vi "Main FPGA 5-axis with 1AxisLimit.vi"() -> ()   [LabVIEW 2013]
uses:
  <vilib>/Motion/MotorControl/_s/nism.interpretControlRegister.stateTransition.ctl
  <vilib>/Platform/TimedLoop/XDataNode/timing_clust.ctl
  <vilib>/Platform/TimedLoop/XDataNode/nitl_modes.ctl
  <vilib>/Platform/TimedLoop/XDataNode/wakeup.ctl
  <vilib>/Motion/MotorControl/_s/nism.digitalInputs.portA.ctl
  <vilib>/rvi/Emulation/niFpgaSctlEmulationGetInTimedLoop.vi
  <vilib>/rvi/Emulation/niFpgaEmulationReportErrorSimple.vi
  <vilib>/rvi/Emulation/niFpgaGetClockAttributes.vi
  <vilib>/rvi/Emulation/niFpgaCriticalErrorInLSC.vi
  Global FPGA.vi
  <vilib>/rvi/eio/common/nirviEmuTemplateMethod_errors.vi
  <vilib>/Motion/SoftMotion/Synchronization/nism.rioScan.generateSyncScan.vi
  <vilib>/rvi/Emulation/niFpgaProcessEmulError.vi
  <vilib>/Motion/MotorControl/_s/nism.interpretControlRegister.indexed.vi
  <vilib>/Motion/MotorControl/_s/nism.generateStatusRegister.indexed.vi
  <vilib>/Motion/MotorControl/_s/nism.mdo.read.positionLoopSyncData.vi
  <vilib>/Motion/MotorControl/_s/nism.mdo.read.splineData.vi
  <vilib>/Motion/MotorControl/_s/nism.splineInterpolation.fxp.3.index.vi
  <vilib>/Motion/MotorControl/_s/nism.mdo.handler.indexed.vi
  <vilib>/Motion/MotorControl/_s/nism.digitalFilter.boolArray.vi
  <vilib>/Motion/MotorControl/_s/nism.interpretDIOControl.portA.single.2.vi
  <vilib>/Motion/MotorControl/_s/nism.generateDIOStatus.portA.single.vi
  <vilib>/Platform/TimedLoop/XDataNode/XDataNode.xnode
  <vilib>/eio/EIONode/EIONode.xnode
  <vilib>/Motion/MotorControl/NI_SoftMotion_MotorControlIP.lvlib
  <vilib>/Platform/TimedLoop/XDataNode/XDNodeRunTimeDep.lvlib
  <vilib>/Motion/SoftMotion/Synchronization/NI_SoftMotion_Synchronization.lvlib
panel:
  in  "DI3":bool
  in  "DI2":bool
  in  "DI1":bool
  in  "DI0":bool
  in  "Home Switch":bool
  in  "Forward Limit":bool
  in  "Reverse Limit":bool
  out "Axis Positions":fxp<+/-,64,32>[](array[numeric])
  in  "STEP or CW? (T=STEP)":bool
  out "Drive Enable":bool[](array[boolean])
  in  "Enable Watchdog":bool
  in  "Pet Watchdog":bool
  in  "Watchdog Timeout Period (ticks)":u64=40000000 format="%.0p"
  out "Watchdog Timed Out?":bool
  out "Time Since Last Pet":u64
  in  "Enable value":bool
  in  "Drive Enable override?":bool
  out "State":T1=enum."Start --> Initializing" caption="state transition"
  in  "Sync Value":bool
  in  "Sync Enable override?":bool
  in  "Invert direction?":bool
  out "Sync is Fault":bool
  out "Sync is Locked":bool
  in  "minimum pulse":u16=40
  # "Synchronization Loop"
  # "Control Status Loop"
  # "Notes: \n1. This VI provides the communication interface between the NI SoftMotion Engine and the LabVIEW FPGA Module. You must compile this VI for a specific FPGA target before use. After compiling, run the VI before running any of the Express VI examples. For information on moving this example to another FPGA target, refer to ni.com/info and enter info code fpgaex.\n\n2. Only use the Reset Axis button if you are unable to communicate with the axis by any other means. This button resets the device state machine and other VIs to a known state. After resetting the axis, switch the NI Scan Engine from Active Mode to Configuration Mode, then back to Active Mode, before attempting to enable the axis."
  # "(These two buttons \nare for testing\npurposes.)"
  # "(These two buttons \nare for testing\npurposes.)"
  # "Step/Direction Loop"
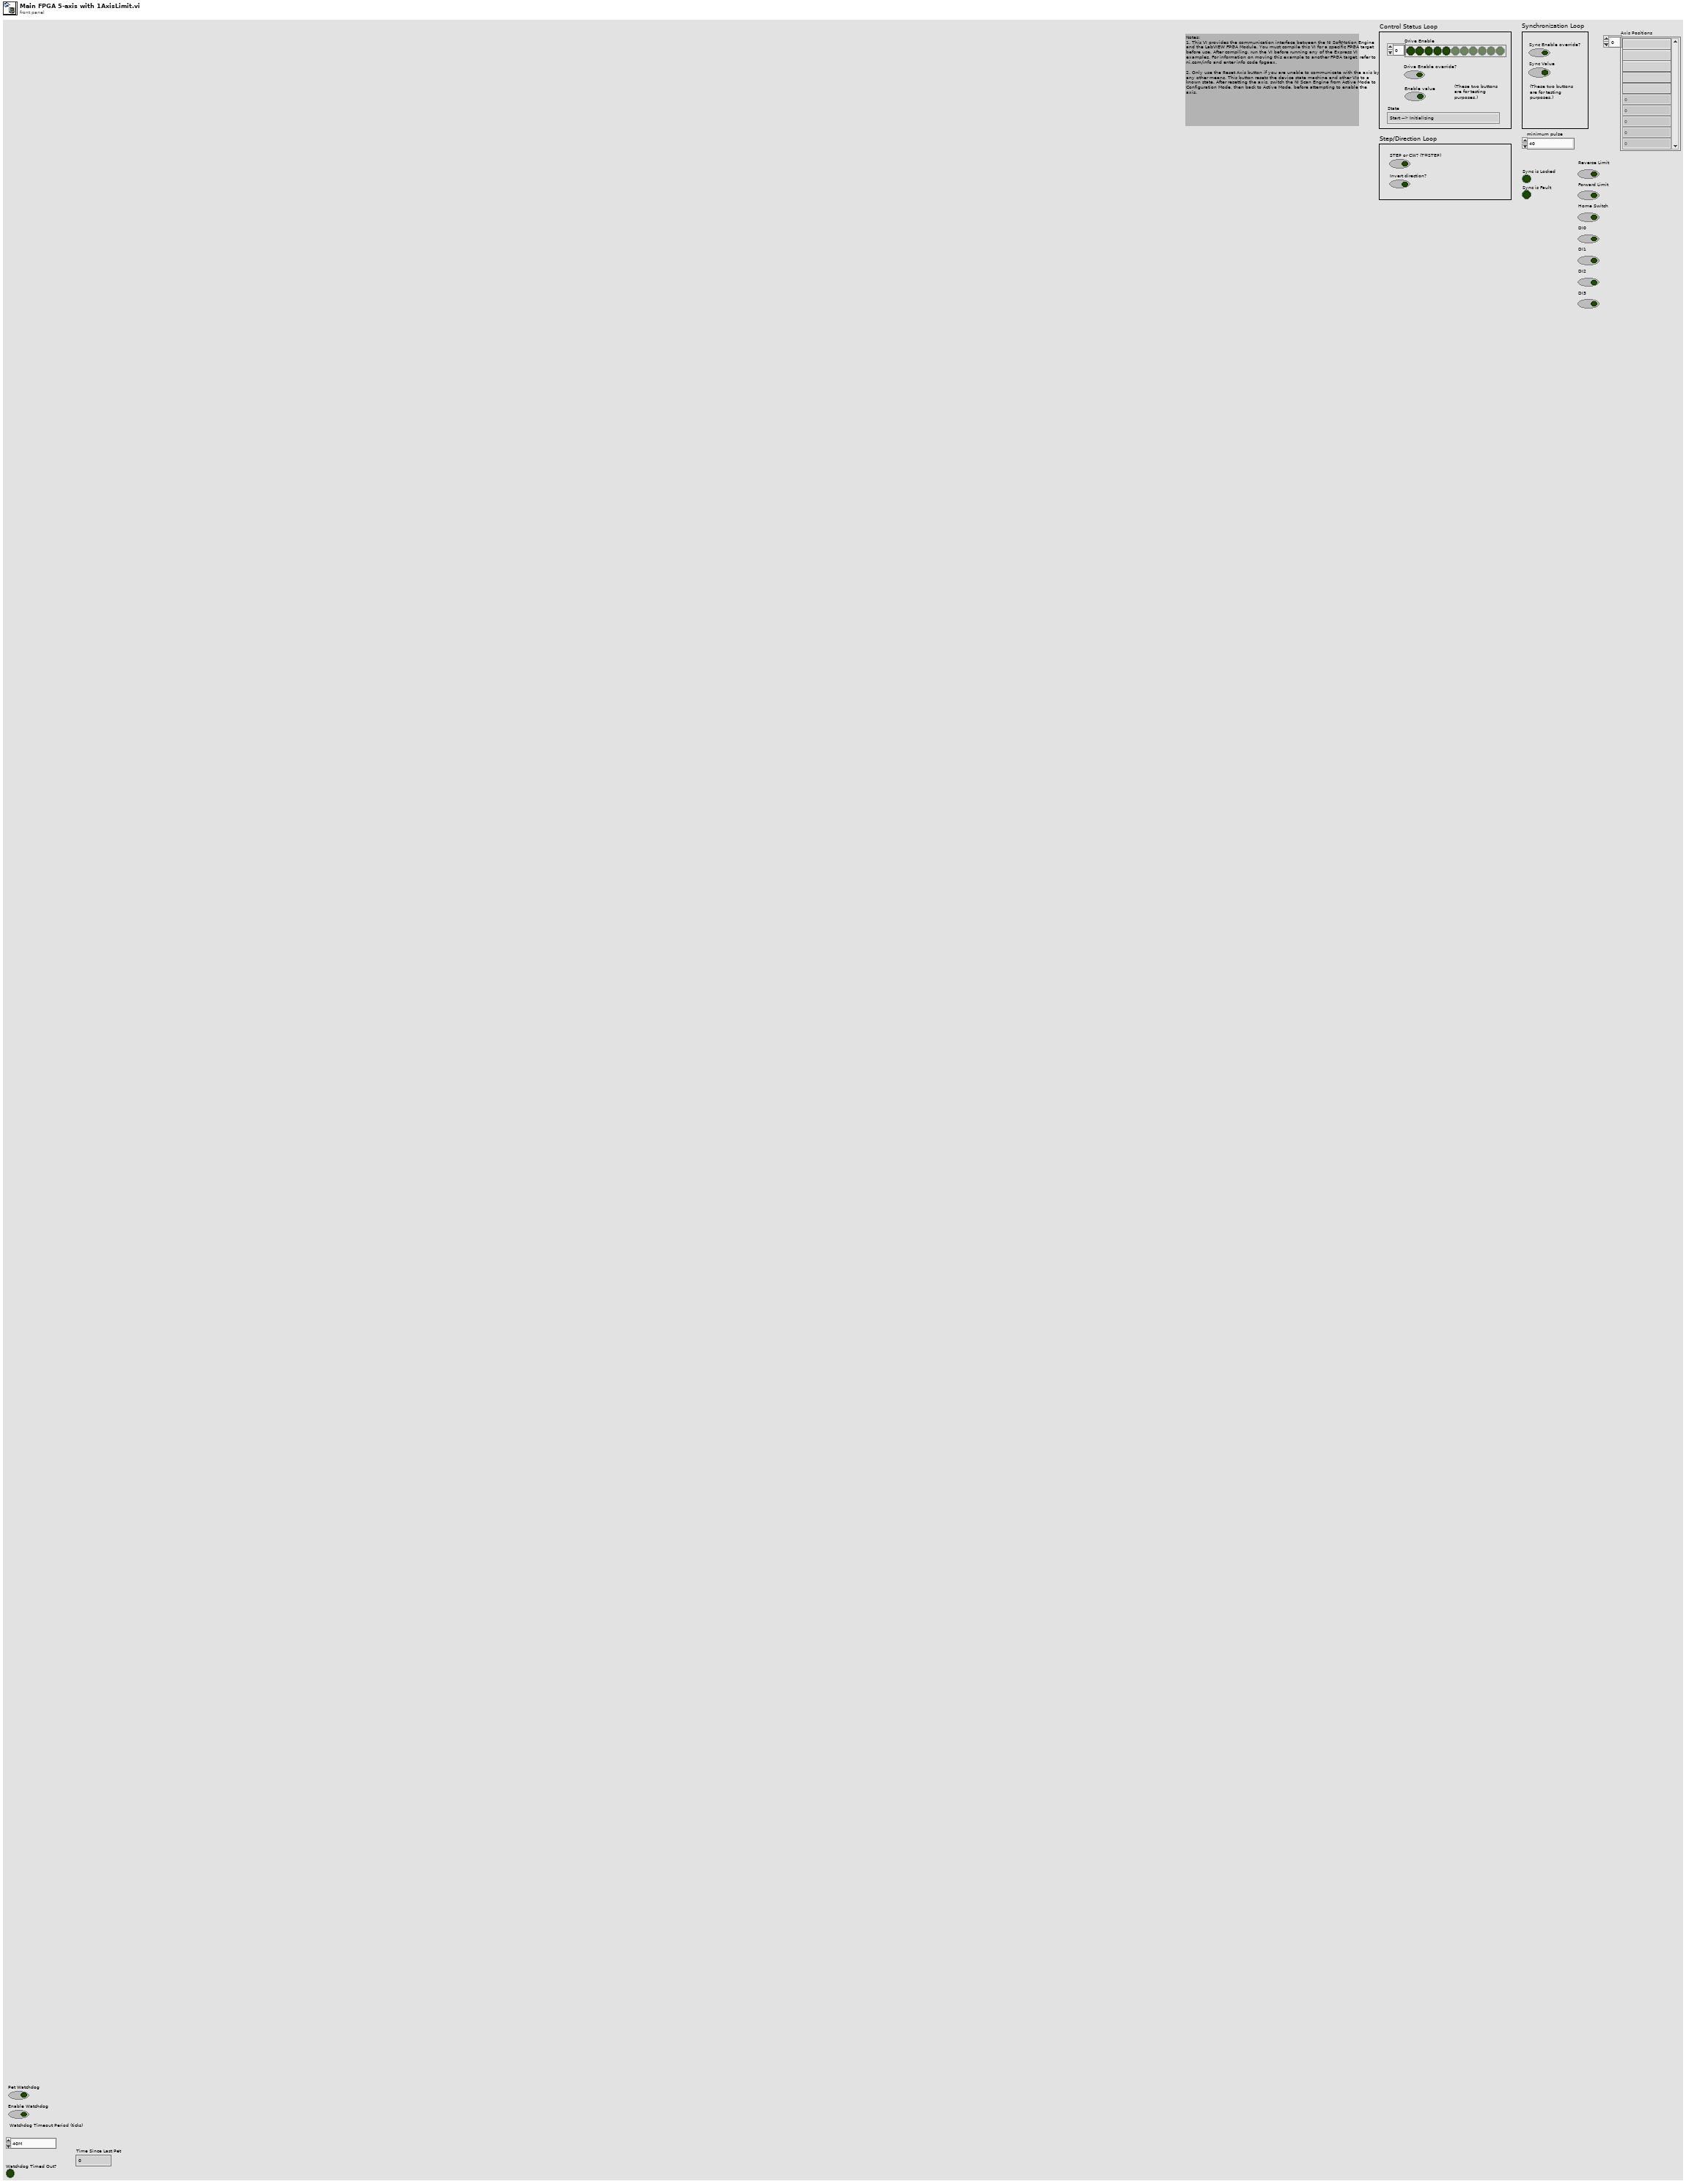
[diagram p1: front panel]
types:
  T1 = typedef "NI_SoftMotion_MotorControlIP.lvlib/nism.interpretControlRegister.stateTransition.ctl" = enum8{"Invalid", "Start --> Initializing", "Initializing --> Disabled", "Disabled --> Ready To Switch On", "Ready To Switch On --> Switched On", "Ready To Switch On --> Disable", "Switched On --> Operation Enable", "Switched On --> Ready To Switch On", "Switched On --> Disabled", "Operation Enable --> Switched On", "Operation Enable --> Ready To Switch On", "Operation Enable --> Disabled", "Fault --> Disabled", "Any --> Fault", "None"}
  T2 = typedef "NI_SoftMotion_MotorControlIP.lvlib/nism.mdo.splineData.ctl" = cluster{"spline type":T3, "traj per/spline per":u16, "spline per/traj per":fxp<+,32,0>}
  T3 = typedef "nism.splineInterpolation.type.ctl" = u16
  T4 = typedef "NI_SoftMotion_Synchronization.lvlib/nism.softmotionScan.timerConfig.ctl" = cluster{"Target Period (clocks)":u16, "Host Period / Target Period":u16}
  T5 = typedef "NI_SoftMotion_Synchronization.lvlib/nism.softmotionScan.timerControl.ctl" = cluster{"SM Scan":bool, "SM Scan Count":u32, "SM Scan Enabled":bool}
  T6 = typedef "XDNodeRunTimeDep.lvlib/timing_clust.ctl" = cluster{"Expected End [f-1]":u64, "Actual End [f-1]":u64, "Finished Late? [f-1]":bool, "Expected End [i-1]":u64, "Actual End [i-1]":u64, "Finished Late? [i-1]":bool, "Expected Start [i]":u64, "Actual Start [i]":u64, "Expected Start [f]":u64, "Actual Start [f]":u64, "Source Name":string, "Structure Name":string, "Period":i64, "Deadline":i64, "Offset":i64, "Start":i64, "Priority":i32, "Timeout":i32, "Mode":T7, "Wakeup Reason":T8, "Error":errorcluster, "Source Type":string, "Secondary Source Type":string, "Global End Time":u64, "Global Start Time":u64, "Frame Duration":u64, "Iteration Duration":u64, "Assigned CPU":i32, "I/O Scan Engine Mode":u32}
  T7 = typedef "XDNodeRunTimeDep.lvlib/nitl_modes.ctl" = enum32{"No Change", "Process missed periods, maintain original phase", "Discard missed periods, maintain original phase", "Process missed periods, ignore original phase", "Discard missed periods, ignore original phase"}
  T8 = typedef "XDNodeRunTimeDep.lvlib/wakeup.ctl" = enum32{"Normal", "Aborted", "Asynchronous wakeup", "Timing source error", "Timed loop error", "Timeout"}
  T9 = typedef "NI_SoftMotion_MotorControlIP.lvlib/nism.digitalInputs.portA.ctl" = cluster{"reverse limit":bool, "forward limit":bool, "home switch":bool, "digital input 0":bool, "digital input 1":bool, "digital input 2":bool, "digital input 3":bool}
  T10 = typedef "NI_SoftMotion_MotorControlIP.lvlib/nism.dio.portA.config.2.ctl" = cluster{"digital filter (us)":u16[], "safe state":enum16{"Low", "High", "No Change"}[]}
  T11 = typedef "NI_SoftMotion_MotorControlIP.lvlib/nism.digitalOutputs.portA.ctl" = cluster{"digital output 0":bool, "digital output 1":bool, "digital output 2":bool, "digital output 3":bool}
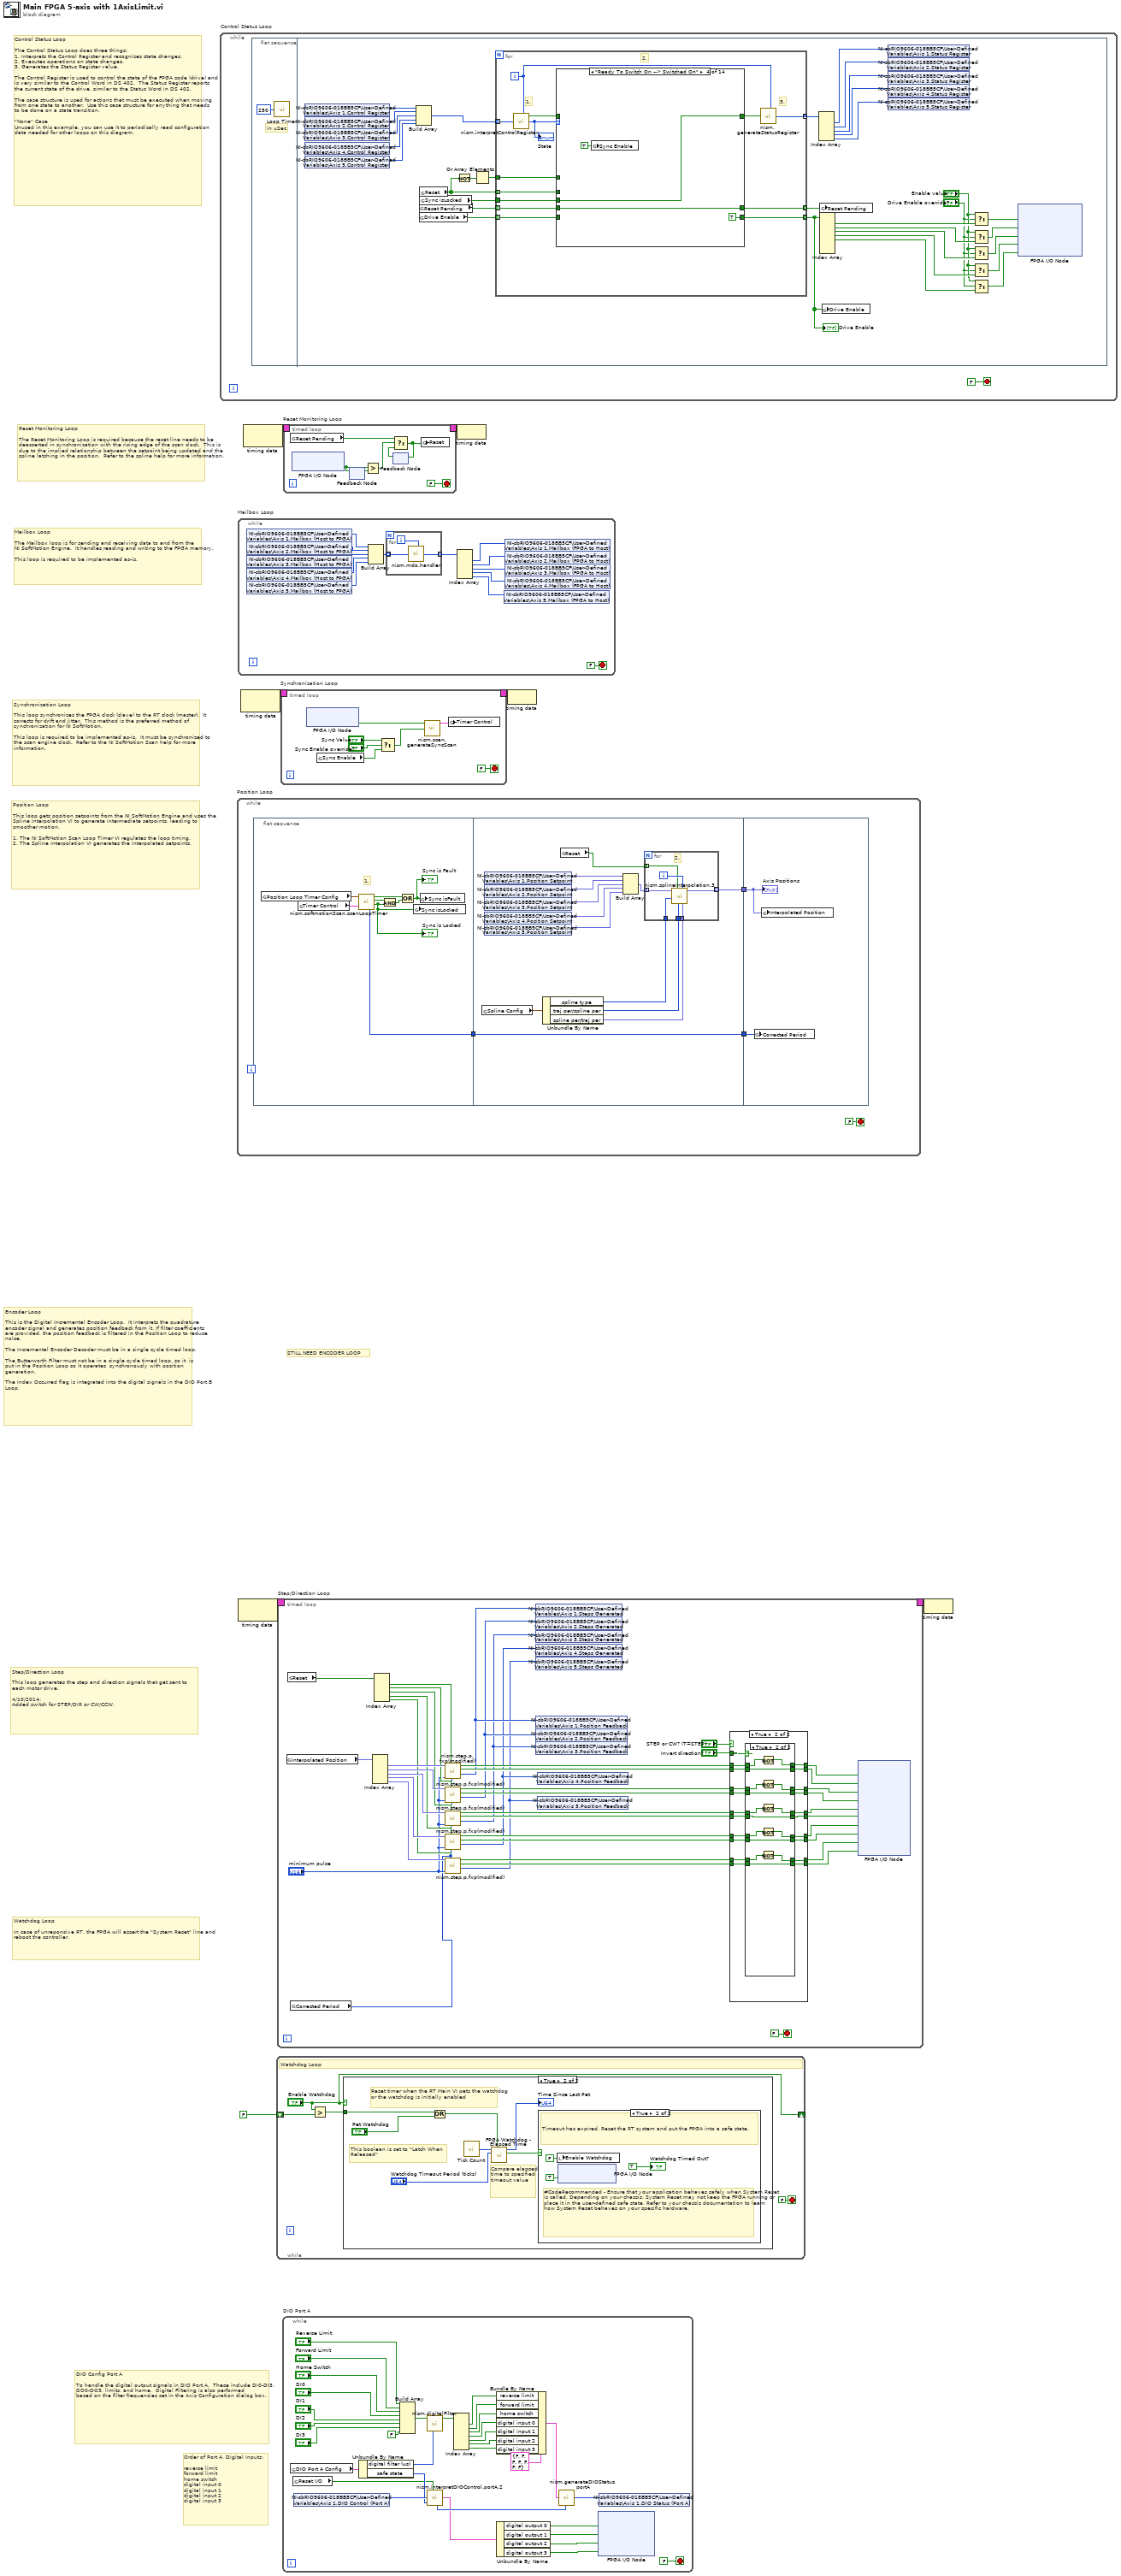
[diagram p0: block diagram]
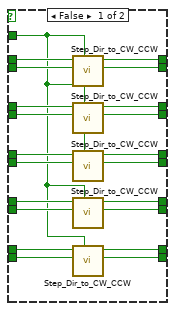
[diagram p4: hidden frame]
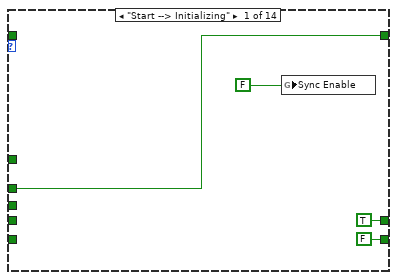
[diagram p6: hidden frame]
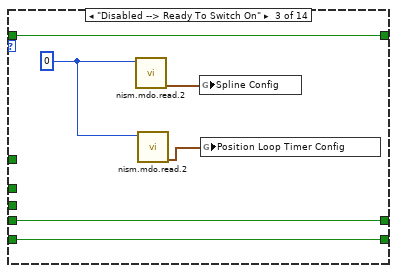
[diagram p8: hidden frame]
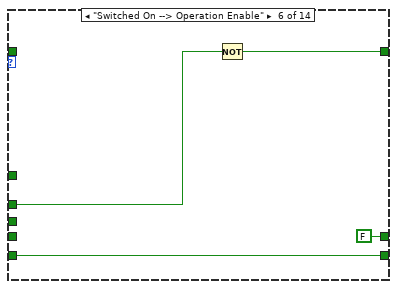
[diagram p10: hidden frame]
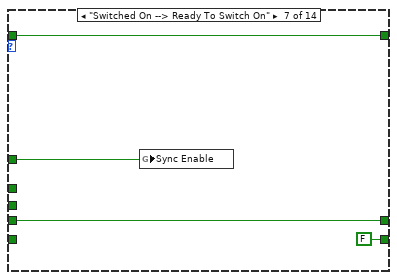
[diagram p11: hidden frame]
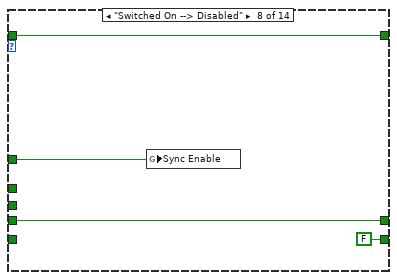
[diagram p12: hidden frame]
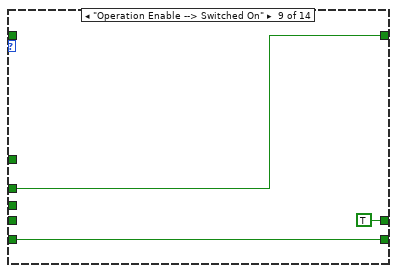
[diagram p13: hidden frame]
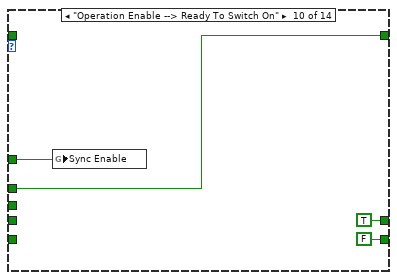
[diagram p14: hidden frame]
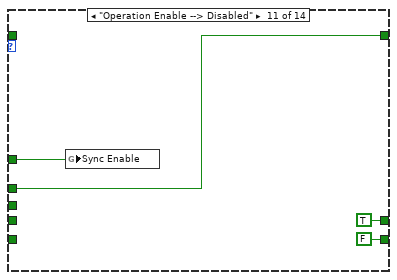
[diagram p15: hidden frame]
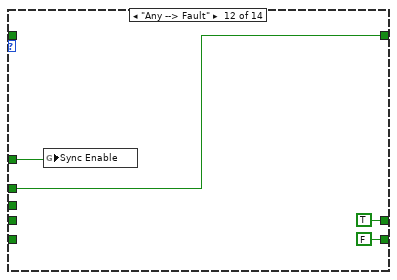
[diagram p16: hidden frame]
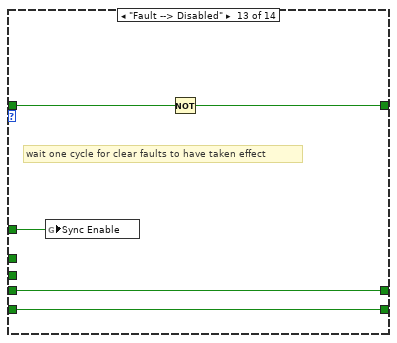
[diagram p17: hidden frame]
diagram:
  # "STILL NEED ENCODER LOOP"
  # "DIO Config Port A\n\nTo handle the digital output signals in DIO Port A.  These include DI0-DI3, DO0-DO3, limits, and home.  Digital Filtering is also performed\nbased on the filter frequencies set in the Axis Configuration dialog box."
  # "Order of Port A, Digital Inputs:\n\nreverse limit\nforward limit\nhome switch\ndigital input 0\ndigital input 1\ndigital input 2\ndigital input 3"
  # "Encoder Loop\n\nThis is the Digital Incremental Encoder Loop.  It interprets the quadrature encoder signal and generates position feedback from it. If filter coefficients are provided, the position feedback is filtered in the Position Loop to reduce noise.\n\nThe Incremental Encoder Decoder must be in a single cycle timed loop.\n\nThe Butterworth Filter must not be in a single cycle timed loop, so it  is\nput in the Position Loop so it operates  synchronously with position generation.\n\nThe Index Occurred flag is integrated into the digital signals in the DIO Port B Loop."
  # "Watchdog Loop\n\nIn case of unreponsive RT, the FPGA will assert the \"System Reset\" line and reboot the controller."
  # "Step/Direction Loop\n\nThis loop generates the step and direction signals that get sent to \neach motor drive.\n\n4/10/2014:\nAdded switch for STEP/DIR or CW/CCW."
  # "Position Loop\n\nThis loop gets position setpoints from the NI SoftMotion Engine and uses the Spline Interpolation VI to generate intermediate setpoints, leading to smoother motion.\n\n1. The NI SoftMotion Scan Loop Timer VI regulates the loop timing. \n2. The Spline Interpolation VI generates the interpolated setpoints."
  # "Synchronization Loop\n\nThis loop synchronizes the FPGA clock (slave) to the RT clock (master).  It corrects for drift and jitter.  This method is the preferred method of synchronization for NI SoftMotion.\n\nThis loop is required to be implemented as-is.  It must be synchronized to the scan engine clock.  Refer to the NI SoftMotion Scan help for more information."
  # "Mailbox Loop\n\nThe Mailbox loop is for sending and receiving data to and from the \nNI SoftMotion Engine.  It handles reading and writing to the FPGA memory.\n\nThis loop is required to be implemented as-is."
  # "Reset Monitoring Loop\n\nThe Reset Monitoring Loop is required because the reset line needs to be deasserted in synchronization with the rising edge of the scan clock.  This is due to the implied relationship between the setpoint being updated and the spline latching in the position.  Refer to the spline help for more information."
  # "Control Status Loop\n\nThe Control Status Loop does three things:\n1. Interprets the Control Register and recognizes state changes.\n2. Executes operations on state changes.\n3. Generates the Status Register value.\n\nThe Control Register is used to control the state of the FPGA code (drive) and is very similar to the Control Word in DS 402.  The Status Register reports the current state of the drive, similar to the Status Word in DS 402.\n\nThe case structure is used for actions that must be executed when moving from one state to another.  Use this case structure for anything that needs to be done on a state transition.\n\n\"None\" Case\nUnused in this example, you can use it to periodically read configuration data needed for other loops on this diagram."
  n1 = while "Control Status Loop" {
    stop <- FALSE stop-if-true
    n2 = flat-sequence {
      frame #0 {
        # "in uSec"
        n3 = call "Loop Timer"("Count(uSec)"=u32 250) -> ()  [unwired: 1 out]
      }
      frame #1 {
        n4 = shared-variable "NI-sbRIO9606-018BB5CF\\User-Defined Variables\\Axis 1.Control Register"() -> (w31:u32)  [unwired: 1 in, 1 out]
        n5 = shared-variable "NI-sbRIO9606-018BB5CF\\User-Defined Variables\\Axis 2.Control Register"() -> (w30:u32)  [unwired: 1 in, 1 out]
        n6 = shared-variable "NI-sbRIO9606-018BB5CF\\User-Defined Variables\\Axis 3.Control Register"() -> (w29:u32)  [unwired: 1 in, 1 out]
        n7 = shared-variable "NI-sbRIO9606-018BB5CF\\User-Defined Variables\\Axis 4.Control Register"() -> (w28:u32)  [unwired: 1 in, 1 out]
        n8 = shared-variable "NI-sbRIO9606-018BB5CF\\User-Defined Variables\\Axis 5.Control Register"() -> (w27:u32)  [unwired: 1 in, 1 out]
        n9 = Build Array(w31, w30, w29, w28, w27) -> (w40:u32[])
        n10 = global read "Global FPGA.vi" "Reset Pending"() -> (w35:bool[])
        n11 = global read "Global FPGA.vi" "Drive Enable"() -> (w34:bool[])
        n12 = global read "Global FPGA.vi" "Reset"() -> (w36:bool[])
        n13 = global read "Global FPGA.vi" "Sync isLocked"() -> (w41:bool)
        n14 = Not(x=w36) -> (.not. x?=w38:bool[])
        n15 = Or Array Elements(Boolean array=w38) -> (logical OR=w37:bool)
        n16 = for {
          tunnel: w36 -> [w49] mode=indexing
          tunnel: w41 -> [w48]
          tunnel: w40 -> [w50] mode=indexing
          tunnel: [w47] -> w32 mode=indexing
          tunnel: [w46] -> w39 mode=indexing
          tunnel: [w45] -> w33 mode=indexing
          tunnel: w37 -> [w44]
          tunnel: w35 -> [w43] mode=indexing
          tunnel: w34 -> [w42] mode=indexing
          i -> [w51]
          # "3."
          # "2."
          # "1."
          n17 = call-poly <vilib>:"nism.interpretControlRegister.vi"("control register"=w50, "axis index"=w51) -> ("transition occurred"=w52:bool, "state transition"=w53:T1)  [unwired: 6 in]
          "State" <- w53
          n18 = case shown="\"Ready To Switch On --> Switched On\"" w53 {
            tunnel: w52 -> [_ w61 w67 _ w74 _ w82 w86 _ _ _ _ w106 _]
            tunnel: [w58 w61 w67 w69 w74 w78 w82 w86 w88 w91 w95 w99 w105 _] -> w54
            tunnel: w49 -> [w58 _ _ _ _ w77 _ _ w88 w91 w95 w99 _ _]
            tunnel: w48 -> [_ _ _ w69 _ _ _ _ _ _ _ _ _ _]
            tunnel: [TRUE ("Write.Reset Pending") w60 w63 w68 w73 FALSE ("Write.Reset Pending") w79 w83 TRUE ("Write.Reset Pending") TRUE ("Write.Reset Pending") TRUE ("Write.Reset Pending") TRUE ("Write.Reset Pending") w103 w108] -> w46
            tunnel: [FALSE ("Write.Drive Enable") w59 w62 TRUE ("Write.Drive Enable") w72 w75 FALSE ("Write.Drive Enable") FALSE ("Write.Drive Enable") w87 FALSE ("Write.Drive Enable") FALSE ("Write.Drive Enable") FALSE ("Write.Drive Enable") w102 w107] -> w45
            tunnel: w44 -> [_ _ _ _ _ _ w80 w84 _ w90 w94 w98 w104 _]
            tunnel: w43 -> [_ w60 w63 w68 w73 _ w79 w83 _ _ _ _ w103 w108]
            tunnel: w42 -> [_ w59 w62 _ w72 w75 _ _ w87 _ _ _ w102 w107]
            frame "Start --> Initializing" {
              n19 = global write "Global FPGA.vi" "Sync Enable"(FALSE ("Sync Enable")) -> ()
            }
            frame "Initializing --> Disabled" {
            }
            frame "Disabled --> Ready To Switch On" {
              w65 = 0 ("axis index")
              n20 = call-poly <vilib>:"nism.mdo.read.2.vi"("axis index"=w65) -> ("spline"=w66:T2)  [unwired: 10 in]
              n21 = call-poly <vilib>:"nism.mdo.read.2.vi"("axis index"=w65) -> ("position loop sync"=w64:T4)  [unwired: 10 in]
              n22 = global write "Global FPGA.vi" "Spline Config"(w66) -> ()
              n23 = global write "Global FPGA.vi" "Position Loop Timer Config"(w64) -> ()
            }
            frame "Ready To Switch On --> Switched On" {
              n24 = global write "Global FPGA.vi" "Sync Enable"(TRUE ("Sync Enable")) -> ()
            }
            frame "Ready To Switch On --> Disable" {
            }
            frame "Switched On --> Operation Enable" {
              n25 = Not(x=w77) -> (.not. x?=w78:bool)
            }
            frame "Switched On --> Ready To Switch On" {
              n26 = global write "Global FPGA.vi" "Sync Enable"(w80) -> ()
            }
            frame "Switched On --> Disabled" {
              n27 = global write "Global FPGA.vi" "Sync Enable"(w84) -> ()
            }
            frame "Operation Enable --> Switched On" {
            }
            frame "Operation Enable --> Ready To Switch On" {
              n28 = global write "Global FPGA.vi" "Sync Enable"(w90) -> ()
            }
            frame "Operation Enable --> Disabled" {
              n29 = global write "Global FPGA.vi" "Sync Enable"(w94) -> ()
            }
            frame "Any --> Fault" {
              n30 = global write "Global FPGA.vi" "Sync Enable"(w98) -> ()
            }
            frame "Fault --> Disabled" {
              # "wait one cycle for clear faults to have taken effect"
              n31 = global write "Global FPGA.vi" "Sync Enable"(w104) -> ()
              n32 = Not(x=w106) -> (.not. x?=w105:bool)
            }
            frame "None", Default {
            }
          }
          n33 = call-poly <vilib>:"nism.generateStatusRegister.vi"("transition success"=w54, "axis index"=w51) -> ("status register"=w47:u32)  [unwired: 7 in]
        }
        "Drive Enable" <- w33
        n34 = Index Array(array=w32) -> (element #1=w26:u32, element #2=w25:u32, element #3=w24:u32, element #4=w23:u32, element #5=w22:u32)  [unwired: 5 in]
        n35 = global write "Global FPGA.vi" "Reset Pending"(w39) -> ()
        n36 = Index Array(array=w33) -> (element #1=w21:bool, element #2=w19:bool, element #3=w17:bool, element #4=w15:bool, element #5=w13:bool)  [unwired: 8 in, 3 out]
        n37 = global write "Global FPGA.vi" "Drive Enable"(w33) -> ()
        n38 = shared-variable "NI-sbRIO9606-018BB5CF\\User-Defined Variables\\Axis 1.Status Register"(w26) -> ()  [unwired: 1 in, 1 out]
        n39 = shared-variable "NI-sbRIO9606-018BB5CF\\User-Defined Variables\\Axis 2.Status Register"(w25) -> ()  [unwired: 1 in, 1 out]
        n40 = shared-variable "NI-sbRIO9606-018BB5CF\\User-Defined Variables\\Axis 3.Status Register"(w24) -> ()  [unwired: 1 in, 1 out]
        n41 = shared-variable "NI-sbRIO9606-018BB5CF\\User-Defined Variables\\Axis 4.Status Register"(w23) -> ()  [unwired: 1 in, 1 out]
        n42 = shared-variable "NI-sbRIO9606-018BB5CF\\User-Defined Variables\\Axis 5.Status Register"(w22) -> ()  [unwired: 1 in, 1 out]
        n43 = Select(t="Enable value", s="Drive Enable override?", f=w21) -> (s? t:f=w20:bool)
        n44 = Select(t="Enable value", s="Drive Enable override?", f=w19) -> (s? t:f=w18:bool)
        n45 = Select(t="Enable value", s="Drive Enable override?", f=w17) -> (s? t:f=w16:bool)
        n46 = Select(t="Enable value", s="Drive Enable override?", f=w15) -> (s? t:f=w14:bool)
        n47 = Select(t="Enable value", s="Drive Enable override?", f=w13) -> (s? t:f=w12:bool)
        n48 = xnode "FPGA I/O Node"("Axis1_Servo On"=w20, "Axis2_Servo On"=w18, "Axis3_Servo On"=w16, "Axis4_Servo On"=w14, "Axis5_Servo On"=w12) -> ()  [unwired: 5 in, 5 out]
      }
    }
  }
  n49 = while "Position Loop" {
    stop <- FALSE stop-if-true
    n50 = flat-sequence {
      tunnel: [w113] -> w109
      tunnel: [w127] -> w111
      tunnel: [w126] -> w110
      tunnel: w109 -> [w126]
      tunnel: w111 -> [w141]
      tunnel: w110 -> [w142]
      frame #0 {
        # "1."
        n51 = global read "Global FPGA.vi" "Position Loop Timer Config"() -> (w115:T4)
        n52 = global read "Global FPGA.vi" "Timer Control"() -> (w114:T5)
        n53 = call <vilib>:"nism.softmotionScan.scanLoopTimer.vi"("Timer Control"=w114, "Timer Config"=w115) -> ("Scan Running?"=w117:bool, "Finished Late?"=w119:bool, "Fault Occurred?"=w120:bool, "Corrected Period"=w113:u16)  [unwired: 5 in, 1 out]
        "Sync is Locked" <- w117
        n54 = Compound Arithmetic op=AND(w119, w117) -> (w118:bool)
        n55 = Compound Arithmetic op=OR(w120, w118) -> (w116:bool)
        "Sync is Fault" <- w116
        n56 = global write "Global FPGA.vi" "Sync isLocked"(w117) -> ()
        n57 = global write "Global FPGA.vi" "Sync isFault"(w116) -> ()
      }
      frame #1 {
        n58 = global read "Global FPGA.vi" "Spline Config"() -> (w129:T2)
        n59 = shared-variable "NI-sbRIO9606-018BB5CF\\User-Defined Variables\\Axis 1.Position Setpoint"() -> (w125:fxp<+/-,64,32>)  [unwired: 1 in, 1 out]
        n60 = shared-variable "NI-sbRIO9606-018BB5CF\\User-Defined Variables\\Axis 2.Position Setpoint"() -> (w124:fxp<+/-,64,32>)  [unwired: 1 in, 1 out]
        n61 = shared-variable "NI-sbRIO9606-018BB5CF\\User-Defined Variables\\Axis 3.Position Setpoint"() -> (w123:fxp<+/-,64,32>)  [unwired: 1 in, 1 out]
        n62 = shared-variable "NI-sbRIO9606-018BB5CF\\User-Defined Variables\\Axis 4.Position Setpoint"() -> (w122:fxp<+/-,64,32>)  [unwired: 1 in, 1 out]
        n63 = shared-variable "NI-sbRIO9606-018BB5CF\\User-Defined Variables\\Axis 5.Position Setpoint"() -> (w121:fxp<+/-,64,32>)  [unwired: 1 in, 1 out]
        n64 = Unbundle By Name(w129) -> ("spline type"=w133:T3, "traj per/spline per"=w132:u16, "spline per/traj per"=w131:fxp<+,32,0>)
        n65 = global read "Global FPGA.vi" "Reset"() -> (w128:bool[])
        n66 = Build Array(w125, w124, w123, w122, w121) -> (w130:fxp<+/-,64,32>[])
        n67 = for {
          tunnel: w133 -> [w140]
          tunnel: w132 -> [w139]
          tunnel: w131 -> [w138]
          tunnel: w128 -> [w135] mode=indexing
          tunnel: w130 -> [w137] mode=indexing
          tunnel: [w134] -> w127 mode=indexing
          i -> [w136]
          # "2."
          n68 = call-poly <vilib>:"nism.splineInterpolation.3.vi"("1 / calls per sample"=w138, "index"=w136, "calls per sample"=w139, "reset"=w135, "spline type"=w140, "x"=w137) -> ("xi"=w134:fxp<+/-,64,32>)  [unwired: 5 in]
        }
      }
      frame #2 {
        n69 = global write "Global FPGA.vi" "Corrected Period"(w142) -> ()
        n70 = global write "Global FPGA.vi" "Interpolated Position"(w141) -> ()
        "Axis Positions" <- w141
      }
    }
  }
  n71 = while "Mailbox Loop" {
    stop <- FALSE stop-if-true
    n72 = shared-variable "NI-sbRIO9606-018BB5CF\\User-Defined Variables\\Axis 1.Mailbox (Host to FPGA)"() -> (w152:u64)  [unwired: 1 in, 1 out]
    n73 = shared-variable "NI-sbRIO9606-018BB5CF\\User-Defined Variables\\Axis 2.Mailbox (Host to FPGA)"() -> (w151:u64)  [unwired: 1 in, 1 out]
    n74 = shared-variable "NI-sbRIO9606-018BB5CF\\User-Defined Variables\\Axis 3.Mailbox (Host to FPGA)"() -> (w150:u64)  [unwired: 1 in, 1 out]
    n75 = shared-variable "NI-sbRIO9606-018BB5CF\\User-Defined Variables\\Axis 4.Mailbox (Host to FPGA)"() -> (w149:u64)  [unwired: 1 in, 1 out]
    n76 = shared-variable "NI-sbRIO9606-018BB5CF\\User-Defined Variables\\Axis 5.Mailbox (Host to FPGA)"() -> (w148:u64)  [unwired: 1 in, 1 out]
    n77 = Build Array(w152, w151, w150, w149, w148) -> (w154:u64[])
    n78 = for {
      tunnel: w154 -> [w158] mode=indexing
      tunnel: [w157] -> w153 mode=indexing
      i -> [w156]
      n79 = call-poly <vilib>:"nism.mdo.handler.vi"("mbox (host to fpga)"=w158, "axis index"=w156) -> ("mbox (fpga to host)"=w157:u64)  [unwired: 7 in]
    }
    n80 = Index Array(array=w153) -> (element #1=w147:u64, element #2=w146:u64, element #3=w145:u64, element #4=w144:u64, element #5=w143:u64)  [unwired: 5 in]
    n81 = shared-variable "NI-sbRIO9606-018BB5CF\\User-Defined Variables\\Axis 5.Mailbox (FPGA to Host)"(w143) -> ()  [unwired: 1 in, 1 out]
    n82 = shared-variable "NI-sbRIO9606-018BB5CF\\User-Defined Variables\\Axis 1.Mailbox (FPGA to Host)"(w147) -> ()  [unwired: 1 in, 1 out]
    n83 = shared-variable "NI-sbRIO9606-018BB5CF\\User-Defined Variables\\Axis 2.Mailbox (FPGA to Host)"(w146) -> ()  [unwired: 1 in, 1 out]
    n84 = shared-variable "NI-sbRIO9606-018BB5CF\\User-Defined Variables\\Axis 3.Mailbox (FPGA to Host)"(w145) -> ()  [unwired: 1 in, 1 out]
    n85 = shared-variable "NI-sbRIO9606-018BB5CF\\User-Defined Variables\\Axis 4.Mailbox (FPGA to Host)"(w144) -> ()  [unwired: 1 in, 1 out]
  }
  n86 = node-c288() -> (w7:T6)  [unwired: 1 in]
  n87 = node-c288() -> (w5:T6)  [unwired: 1 in]
  n88 = node-c288() -> (w3:T6)  [unwired: 1 in]
  n89 = while "RT Watchdog Loop" {
    shift-right: ["Enable Watchdog"] -> _
    shift-left: FALSE ("Enable RT Watchdog") -> [w162]
    stop <- FALSE stop-if-true
    # "Watchdog Loop"
    n90 = Greater?(x="Enable Watchdog", y=w162) -> (0:w159:bool)
    n91 = case shown="True" "Enable Watchdog" {
      tunnel: w159 -> [_ w165]
      frame False {
        # "This loop has to be explicitly enabled from the RT Main VI.  This reduces the possiblity of an endless reboot cycle."
      }
      frame True {
        # "This boolean is set to \"Latch When Released\""
        # "Compare elapsed time to specified timeout value"
        # "Reset timer when the RT Main VI pets the watchdog or the watchdog is initially enabled"
        n92 = Or(x=w165, y="Pet Watchdog") -> (x .or. y?=w164:bool)
        n93 = call "Tick Count"() -> ("Tick Count(Ticks)"=w168:u32)
        n94 = call "FPGA Watchdog - Elapsed Time.vi"("Reset"=w164, "Timeout Period"="Watchdog Timeout Period (ticks)", "Current Time"=w168) -> ("Timeout"=w163:bool, "Elapsed Time"=→"Time Since Last Pet":u64)  [unwired: 7 in]
        n95 = case shown="True" w163 {
          frame False {
            # "Timeout has not expired."
          }
          frame True {
            # "#CodeRecommended - Ensure that your application behaves safely when System Reset is called. Depending on your chassis, System Reset may not keep the FPGA running or place it in the user-defined safe state. Refer to your chassis documentation to learn how System Reset behaves on your specific hardware."
            # "Timeout has expired. Reset the RT system and put the FPGA into a safe state."
            n96 = local write "Enable Watchdog"(FALSE ("Enable RT Watchdog")) -> ()
            n97 = xnode "FPGA I/O Node"("System Reset"=TRUE ("RT Reset on Watchdog Failure?")) -> ()  [unwired: 1 in, 1 out]
            "Watchdog Timed Out?" <- TRUE ("Watchdog Timed Out?")
          }
        }
      }
    }
  }
  n98 = timed-loop "Step/Direction Loop" {
    timing: w7 -> [_]
    timing-out: [_] -> w6
    stop <- FALSE stop-if-true
    n99 = global read "Global FPGA.vi" "Interpolated Position"() -> (w213:fxp<+/-,64,32>[])
    n100 = global read "Global FPGA.vi" "Reset"() -> (w207:bool[])
    n101 = global read "Global FPGA.vi" "Corrected Period"() -> (w173:u16)
    n102 = Index Array(array=w213) -> (element #1=w212:fxp<+/-,64,32>, element #2=w211:fxp<+/-,64,32>, element #3=w210:fxp<+/-,64,32>, element #4=w209:fxp<+/-,64,32>, element #5=w208:fxp<+/-,64,32>)  [unwired: 5 in]
    n103 = Index Array(array=w207) -> (element #1=w206:bool, element #2=w205:bool, element #3=w204:bool, element #4=w203:bool, element #5=w202:bool)  [unwired: 5 in]
    n104 = call "nism.step.p.fxp(modified).vi"("calls per sample"=w173, "reset"=w206, "minimum pulse"="minimum pulse", "position setpoint"=w212) -> ("steps generated"=w178:i32, "step"=w200:bool, "direction"=w201:bool)  [unwired: 4 in, 1 out]
    n105 = call "nism.step.p.fxp(modified).vi"("calls per sample"=w173, "reset"=w205, "minimum pulse"="minimum pulse", "position setpoint"=w211) -> ("steps generated"=w177:i32, "step"=w198:bool, "direction"=w199:bool)  [unwired: 4 in, 1 out]
    n106 = call "nism.step.p.fxp(modified).vi"("calls per sample"=w173, "reset"=w204, "minimum pulse"="minimum pulse", "position setpoint"=w210) -> ("steps generated"=w176:i32, "step"=w196:bool, "direction"=w197:bool)  [unwired: 4 in, 1 out]
    n107 = call "nism.step.p.fxp(modified).vi"("calls per sample"=w173, "reset"=w203, "minimum pulse"="minimum pulse", "position setpoint"=w209) -> ("steps generated"=w175:i32, "step"=w194:bool, "direction"=w195:bool)  [unwired: 4 in, 1 out]
    n108 = call "nism.step.p.fxp(modified).vi"("calls per sample"=w173, "reset"=w202, "minimum pulse"="minimum pulse", "position setpoint"=w208) -> ("steps generated"=w174:i32, "step"=w192:bool, "direction"=w193:bool)  [unwired: 4 in, 1 out]
    n109 = shared-variable "NI-sbRIO9606-018BB5CF\\User-Defined Variables\\Axis 1.Steps Generated"(w178) -> ()  [unwired: 1 in, 1 out]
    n110 = shared-variable "NI-sbRIO9606-018BB5CF\\User-Defined Variables\\Axis 2.Steps Generated"(w177) -> ()  [unwired: 1 in, 1 out]
    n111 = shared-variable "NI-sbRIO9606-018BB5CF\\User-Defined Variables\\Axis 3.Steps Generated"(w176) -> ()  [unwired: 1 in, 1 out]
    n112 = shared-variable "NI-sbRIO9606-018BB5CF\\User-Defined Variables\\Axis 4.Steps Generated"(w175) -> ()  [unwired: 1 in, 1 out]
    n113 = shared-variable "NI-sbRIO9606-018BB5CF\\User-Defined Variables\\Axis 5.Steps Generated"(w174) -> ()  [unwired: 1 in, 1 out]
    n114 = shared-variable "NI-sbRIO9606-018BB5CF\\User-Defined Variables\\Axis 1.Position Feedback"(w178) -> ()  [unwired: 1 in, 1 out]
    n115 = shared-variable "NI-sbRIO9606-018BB5CF\\User-Defined Variables\\Axis 2.Position Feedback"(w177) -> ()  [unwired: 1 in, 1 out]
    n116 = shared-variable "NI-sbRIO9606-018BB5CF\\User-Defined Variables\\Axis 3.Position Feedback"(w176) -> ()  [unwired: 1 in, 1 out]
    n117 = shared-variable "NI-sbRIO9606-018BB5CF\\User-Defined Variables\\Axis 4.Position Feedback"(w175) -> ()  [unwired: 1 in, 1 out]
    n118 = shared-variable "NI-sbRIO9606-018BB5CF\\User-Defined Variables\\Axis 5.Position Feedback"(w174) -> ()  [unwired: 1 in, 1 out]
    n119 = case shown="True" "STEP or CW? (T=STEP)" {
      tunnel: w201 -> [w235 w255]
      tunnel: w200 -> [w234 w245]
      tunnel: w199 -> [w233 w253]
      tunnel: w198 -> [w232 w243]
      tunnel: w197 -> [w231 w251]
      tunnel: w196 -> [w230 w241]
      tunnel: w195 -> [w229 w249]
      tunnel: w194 -> [w228 w239]
      tunnel: w193 -> [w227 w247]
      tunnel: w192 -> [w226 w237]
      tunnel: "Invert direction?" -> [w215 w256]
      tunnel: [w225 w254] -> w190
      tunnel: [w224 w244] -> w181
      tunnel: [w223 w252] -> w189
      tunnel: [w222 w242] -> w188
      tunnel: [w221 w250] -> w187
      tunnel: [w220 w240] -> w186
      tunnel: [w219 w248] -> w185
      tunnel: [w218 w238] -> w184
      tunnel: [w217 w246] -> w183
      tunnel: [w216 w236] -> w182
      frame False {
        n120 = call "Step_Dir_to_CW_CCW.vi"("invert"=w215, "step"=w234, "direction"=w235) -> ("CCW"=w224:bool, "CW"=w225:bool)  [unwired: 7 in]
        n121 = call "Step_Dir_to_CW_CCW.vi"("invert"=w215, "step"=w232, "direction"=w233) -> ("CCW"=w222:bool, "CW"=w223:bool)  [unwired: 7 in]
        n122 = call "Step_Dir_to_CW_CCW.vi"("invert"=w215, "step"=w230, "direction"=w231) -> ("CCW"=w220:bool, "CW"=w221:bool)  [unwired: 7 in]
        n123 = call "Step_Dir_to_CW_CCW.vi"("invert"=w215, "step"=w228, "direction"=w229) -> ("CCW"=w218:bool, "CW"=w219:bool)  [unwired: 7 in]
        n124 = call "Step_Dir_to_CW_CCW.vi"("invert"=w215, "step"=w226, "direction"=w227) -> ("CCW"=w216:bool, "CW"=w217:bool)  [unwired: 7 in]
      }
      frame True {
        n125 = case shown="True" w256 {
          tunnel: w255 -> [w266 w281]
          tunnel: [w266 w280] -> w254
          tunnel: w253 -> [w264 w279]
          tunnel: [w264 w278] -> w252
          tunnel: w251 -> [w262 w277]
          tunnel: [w262 w276] -> w250
          tunnel: w249 -> [w260 w275]
          tunnel: [w260 w274] -> w248
          tunnel: w247 -> [w258 w273]
          tunnel: [w258 w272] -> w246
          tunnel: w245 -> [w265 w271]
          tunnel: [w265 w271] -> w244
          tunnel: w243 -> [w263 w270]
          tunnel: [w263 w270] -> w242
          tunnel: w241 -> [w261 w269]
          tunnel: [w261 w269] -> w240
          tunnel: w239 -> [w259 w268]
          tunnel: [w259 w268] -> w238
          tunnel: w237 -> [w257 w267]
          tunnel: [w257 w267] -> w236
          frame False {
          }
          frame True {
            n126 = Not(x=w281) -> (.not. x?=w280:bool)
            n127 = Not(x=w279) -> (.not. x?=w278:bool)
            n128 = Not(x=w277) -> (.not. x?=w276:bool)
            n129 = Not(x=w275) -> (.not. x?=w274:bool)
            n130 = Not(x=w273) -> (.not. x?=w272:bool)
          }
        }
      }
    }
    n131 = xnode "FPGA I/O Node"("Axis1_CW"=w190, "Axis1_CCW"=w181, "Axis2_CW"=w189, "Axis2_CCW"=w188, "Axis3_CW"=w187, "Axis3_CCW"=w186, "Axis4_CW"=w185, "Axis4_CCW"=w184, "Axis5_CW"=w183, "Axis5_CCW"=w182) -> ()  [unwired: 10 in, 10 out]
  }
  n132 = timed-loop "Synchronization Loop" {
    timing: w5 -> [_]
    timing-out: [_] -> w4
    stop <- FALSE stop-if-true
    n133 = xnode "FPGA I/O Node"() -> ("Scan Clock"=w288:bool)  [unwired: 1 in, 1 out]
    n134 = global read "Global FPGA.vi" "Sync Enable"() -> (w287:bool)
    n135 = Select(t="Sync Value", s="Sync Enable override?", f=w287) -> (s? t:f=w284:bool)
    n136 = call-poly <vilib>:"nism.scan.generateSyncScan.vi"("Scan Enable?"=w284, "Scan Clock"=w288) -> ("Timer Control"=w289:T5)  [unwired: 3 in]
    n137 = global write "Global FPGA.vi" "Timer Control"(w289) -> ()
  }
  n138 = while "DIO Port A" {
    stop <- FALSE stop-if-true
    n139 = global read "Global FPGA.vi" "DIO Port A Config"() -> (w302:T10)
    n140 = global read "Global FPGA.vi" "Reset I/O"() -> (w300:bool)
    n141 = shared-variable "NI-sbRIO9606-018BB5CF\\User-Defined Variables\\Axis 1.DIO Control (Port A)"() -> (w322:u32)  [unwired: 1 in, 1 out]
    n142 = Unbundle By Name(w302) -> ("digital filter (us)"=w316:u16[], "safe state"=w301:enum16{"Low", "High", "No Change"}[])
    n143 = Build Array("Reverse Limit", "Forward Limit", "Home Switch", "DI0", "DI1", "DI2", "DI3", FALSE ("element")) -> (w318:bool[])
    n144 = call-poly <vilib>:"nism.digitalFilter.vi"("filter value (us)"=w316, "input signal"=w318) -> ("output signal"=w315:bool[])  [unwired: 9 in]
    n145 = call-poly <vilib>:"nism.interpretDIOControl.portA.2.vi"("reset"=w300, "dio control(port a)"=w322, "safe state"=w301) -> ("digital outputs"=w321:T11, "reset latches"=w324:u8)  [unwired: 5 in]
    n146 = Index Array(array=w315) -> (element #1=w314:bool, element #2=w313:bool, element #3=w312:bool, element #4=w311:bool, element #5=w310:bool, element #6=w309:bool, element #7=w308:bool)  [unwired: 7 in]
    n147 = Bundle By Name(cluster=T9 {"reverse limit"=FALSE, "forward limit"=FALSE, "home switch"=FALSE, "digital input 0"=FALSE, "digital input 1"=FALSE, "digital input 2"=FALSE, "digital input 3"=FALSE} ("$(driveInterface.digitalInputs.shortName)"), "reverse limit"=w314, "forward limit"=w313, "home switch"=w312, "digital input 0"=w311, "digital input 1"=w310, "digital input 2"=w309, "digital input 3"=w308) -> (w319:T9)
    n148 = Unbundle By Name(w321) -> ("digital output 0"=w306:bool, "digital output 1"=w305:bool, "digital output 2"=w304:bool, "digital output 3"=w303:bool)
    n149 = call-poly <vilib>:"nism.generateDIOStatus.portA.vi"("digital inputs"=w319, "reset latches"=w324) -> ("dio status(port a)"=w323:u32)  [unwired: 7 in]
    n150 = xnode "FPGA I/O Node"("FPGA LED"=w306, "RMC/DIO21"=w305, "RMC/DIO22"=w304, "RMC/DIO23"=w303) -> ()  [unwired: 4 in, 4 out]
    n151 = shared-variable "NI-sbRIO9606-018BB5CF\\User-Defined Variables\\Axis 1.DIO Status (Port A)"(w323) -> ()  [unwired: 1 in, 1 out]
  }
  n152 = timed-loop "Reset Monitoring Loop" {
    timing: w3 -> [_]
    timing-out: [_] -> w2
    stop <- FALSE stop-if-true
    n153 = global read "Global FPGA.vi" "Reset Pending"() -> (w327:bool[])
    n154 = xnode "FPGA I/O Node"() -> ("Scan Clock"=w326:bool)  [unwired: 1 in, 1 out]
    n155 = feedback-in #1(w326) -> ()
    n156 = feedback #1() -> (w325:bool)  [unwired: 1 in]
    n157 = Greater?(x=w326, y=w325) -> (0:w331:bool)
    n158 = feedback #2() -> (w330:bool[])  [unwired: 1 in]
    n159 = Select(t=w327, s=w331, f=w330) -> (s? t:f=w328:bool[])
    n160 = feedback-in #2(w328) -> ()
    n161 = global write "Global FPGA.vi" "Reset"(w328) -> ()
  }
  n162 = node-c288(w2) -> ()
  n163 = node-c288(w4) -> ()
  n164 = node-c288(w6) -> ()
